vi "CPP_WhiteNoiseGenerator.vi"() -> ()   [LabVIEW 2016]
uses:
  <vilib>/sound2/lvsound2.llb/Sound Data Format.ctl
  <vilib>/sound2/lvsound2.llb/Sampling Mode.ctl
  <vilib>/Analysis/3filter.llb/Filter Passband Type.ctl
  Globals/Meas_global.vi
  Plug in sub vis/CPP_TubingCompensation/WhiteNoise/WhiteNoiseGlobal.vi
  <vilib>/Analysis/3filter.llb/Butterworth Filter (DBL).vi
  <vilib>/sound2/lvsound2.llb/Sound Output Write (DBL Single).vi
  <vilib>/measure/NI_MABase.lvlib
  <vilib>/Analysis/NI_AALBase.lvlib
panel:
  in  "Device ID":u32
  in  "Amplitude":dbl=1.0
  in  "Cutoff (Hz)":dbl=1000.0
  in  "Overproduce":dbl=1.2
  out "Duration (s)":dbl=16.0
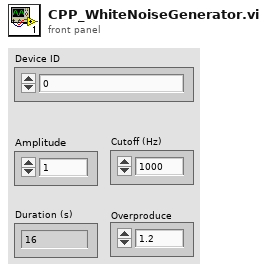
[diagram p1: front panel]
types:
  T1 = typedef "Post_Process.ctl" = enum16{"Take New Data", "Post Process Raw Data File"}
  T2 = typedef "NI_AALBase.lvlib/Filter Passband Type.ctl" = enum32{"Lowpass", "Highpass", "Bandpass", "Bandstop"}
  T3 = typedef "Sampling Mode.ctl" = i32
  T4 = typedef "Sound Data Format.ctl" = cluster{"sample rate (S/s)":dbl, "number of channels":i32, "bits per sample":i32}
  T5 = typedef "Sound Output Task ID.ctl" = u32
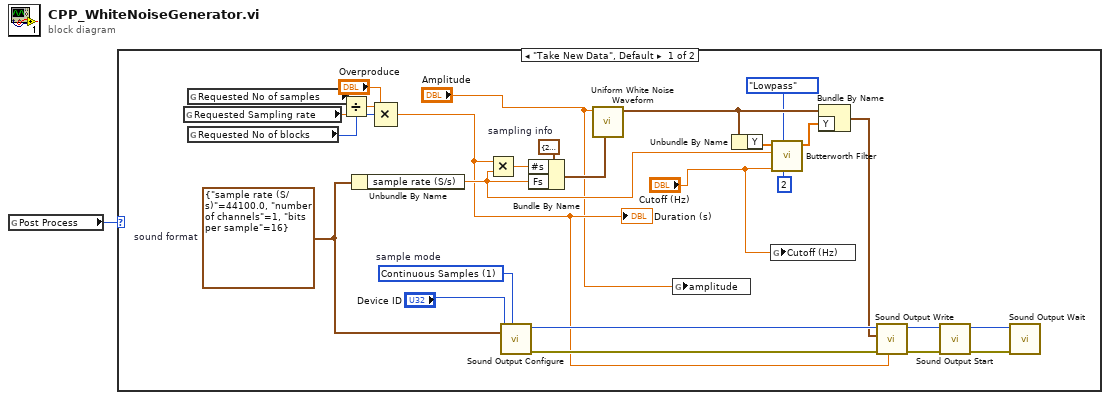
[diagram p0: block diagram]
diagram:
  n1 = global read "Meas_global.vi" "Post Process"() -> (w1:T1)
  n2 = case shown="\"Take New Data\", Default" w1 {
    frame "Take New Data", Default {
      w23 = T3 1 items=["Finite Samples", "Continuous Samples"]  # sample mode
      w25 = T4 {"sample rate (S/s)"=44100.0, "number of channels"=1, "bits per sample"=16}  # sound format
      w27 = cluster{"Fs":dbl, "#s":dbl} {"Fs"=22050.0, "#s"=22050.0}  # sampling info
      n3 = global read "Meas_global.vi" "Requested Sampling rate"() -> (w13:dbl)
      n4 = global read "Meas_global.vi" "Requested No of samples"() -> (w14:i32)
      n5 = global read "Meas_global.vi" "Requested No of blocks"() -> (w11:i32)
      n6 = Divide(x=w14, y=w13) -> (x/y=w12:dbl)
      n7 = Unbundle By Name(w25) -> ("sample rate (S/s)"=w19:dbl)
      n8 = Compound Arithmetic op=MULTIPLY(w12, w11, "Overproduce") -> (w9:dbl)
      "Duration (s)" <- w9
      n9 = Multiply(x=w9, y=w19) -> (x*y=w24:dbl)
      n10 = call <vilib>:"Sound Output Configure.vi"("sample mode"=w23, "sound format"=w25, "device ID"="Device ID") -> ("error out"=w28:errorcluster, "task ID"=w22:T5)  [unwired: 7 in]
      n11 = Bundle By Name(cluster=w27, "#s"=w24, "Fs"=w19) -> (w26:cluster{"Fs":dbl, "#s":dbl})
      n12 = call <vilib>:"Uniform White Noise Waveform.vi"("sampling info"=w26, "amplitude"="Amplitude") -> ("signal out"=w20:waveform(dbl))  [unwired: 8 in, 1 out]
      n13 = global write "WhiteNoiseGlobal.vi" "amplitude"("Amplitude") -> ()
      n14 = Unbundle By Name(w20) -> ("Y"=w17:dbl[])
      n15 = global write "WhiteNoiseGlobal.vi" "Cutoff (Hz)"("Cutoff (Hz)") -> ()
      n16 = call-poly <vilib>:"Butterworth Filter.vi"("order"=2, "filter type"=Filter_Passband_Type."Lowpass", "low cutoff freq: fl"="Cutoff (Hz)", "sampling freq: fs"=w19, "X"=w17) -> ("Filtered X"=w21:dbl[])  [unwired: 3 in, 1 out]
      n17 = Bundle By Name(cluster=w20, "Y"=w21) -> (w18:waveform(dbl))
      n18 = call-poly <vilib>:"Sound Output Write.vi"("timeout (sec)"=w9, "error in (no error)"=w28, "data"=w18, "task ID"=w22) -> ("error out"=w5:errorcluster, "task ID out"=w3:T5)  [unwired: 6 in]
      n19 = call <vilib>:"Sound Output Start.vi"("error in (no error)"=w5, "task ID"=w3) -> ("error out"=w4:errorcluster, "task ID out"=w2:T5)  [unwired: 8 in]
      n20 = call <vilib>:"Sound Output Wait.vi"("error in (no error)"=w4, "task ID"=w2) -> ()  [unwired: 8 in, 2 out]
    }
    frame "Post Process Raw Data File" {
    }
  }
